vi "Model Initial Values - Add Inport RTM.vi"(8 "error in (no error)":errorcluster, 11 "Node Ptr":u64 format="%.0x") -> (0 "error out":errorcluster)   [LabVIEW 2011, in "Model Initial Values Custom Device.lvlib"]
uses:
  Model Initial Values Custom Device.lvlib
  <vilib>/NI Veristand/Custom Device API/Custom Device Item Ref.ctl
  NationalInstruments.VeriStand.SystemStorage
  Model Initial Values - Global.vi
  <vilib>/NI Veristand/Custom Device API/Get Item Property (Dependent Node Pointer).vi
  <vilib>/NI Veristand/Custom Device API/Set Item Property (Double Array).vi
  <vilib>/NI Veristand/Custom Device API/Set Item Property (String Array).vi
  <vilib>/NI Veristand/Custom Device API/Custom Device API.lvlib
  <vilib>/NI Veristand/Custom Device Tools/Custom Device Utility Library/Custom Device Utility Library.lvlib
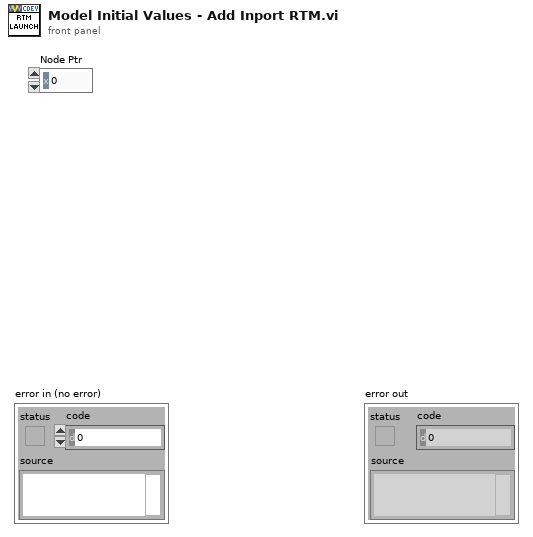
[diagram p1: front panel]
types:
  T1 = typedef "Custom Device API.lvlib/Custom Device Item Ref.ctl" = u64
  T2 = cluster{"MultipleSelection":bool, "ShowCheckBox":bool}
  T3 = typedef "Custom Device API.lvlib/Custom Device Item Info.ctl" = cluster{"Name":string, "Is Channel":bool, "GUID":string}
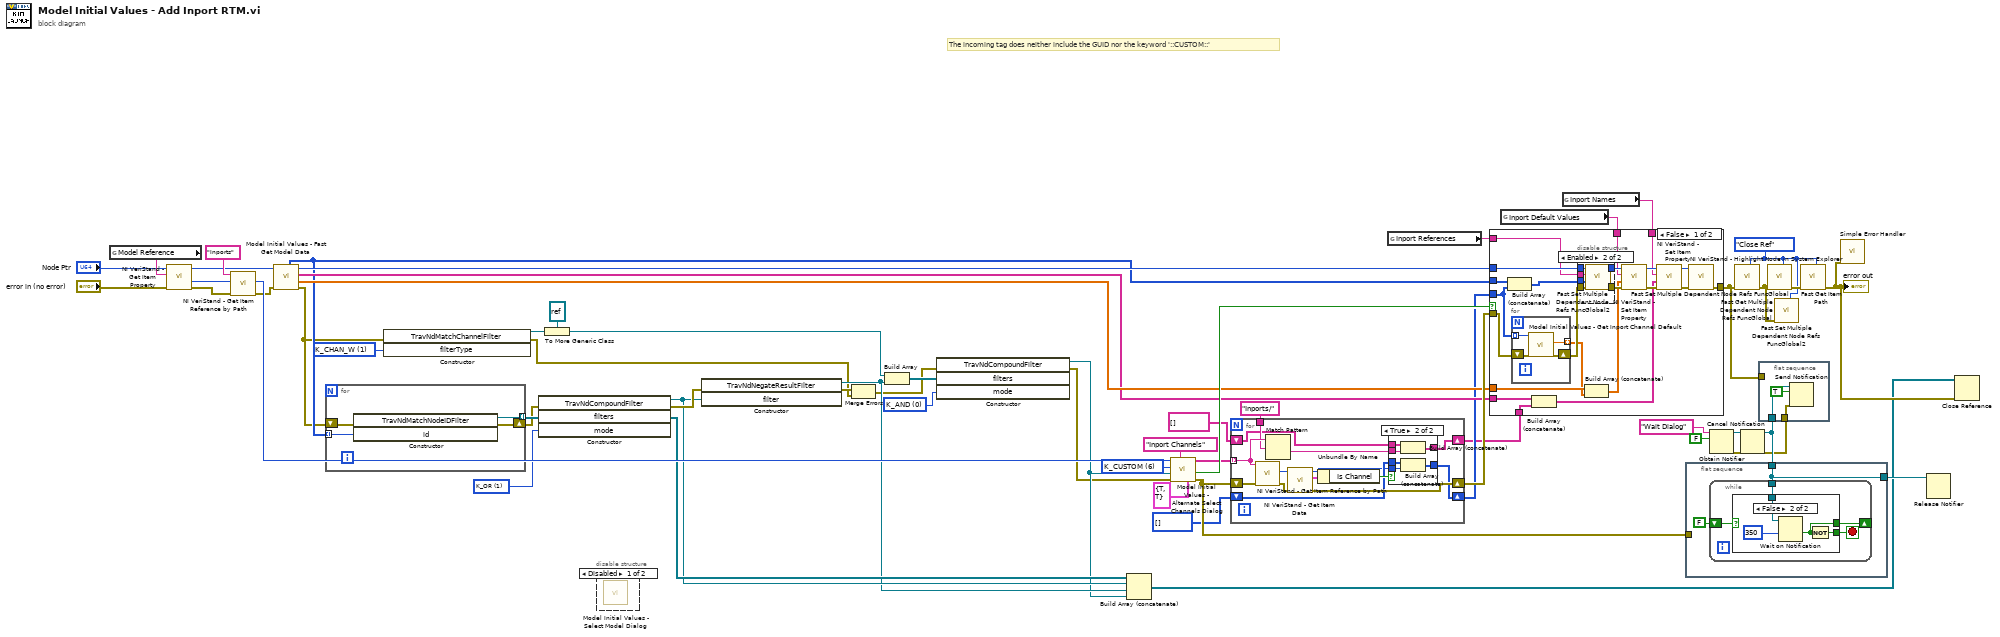
[diagram p0: block diagram]
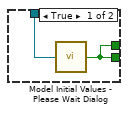
[diagram p3: hidden frame]
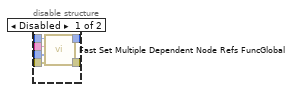
[diagram p5: hidden frame]
diagram:
  w13 = 0 items=["K_AND", "K_OR"] ("mode")
  w14 = u8 1 items=["K_CHAN_R", "K_CHAN_W", "K_CHAN_VOLT", "K_CHAN_FAULT"] ("filterType")
  w28 = 1 items=["K_AND", "K_OR"] ("mode")
  w2 = enum16{"Open or Add", "Close Ref"}."Close Ref" ("Action")
  w51 = u8 6 items=["K_CHAN_R", "K_CHAN_W", "K_CHAN_RW", "K_CHAN_VOLT", "K_CHAN_FAULT", "K_ALL", "K_CUSTOM"] ("Filter")
  # "The incoming tag does neither include the GUID nor the keyword '::CUSTOM::'"
  n1 = global read "Model Initial Values - Global.vi" "Model Reference"() -> (w59:string)
  n2 = call-poly <vilib>:"NI VeriStand - Get Item Property.vi"("error in (no error)"="error in (no error)", "Property Name"=w59, "Item Ref in"="Node Ptr") -> ("error out"=w55:errorcluster, "Dependent Node Ref"=w56:T1, "Item Ref out"=w42:T1)  [unwired: 5 in, 1 out]
  n3 = call <vilib>:"NI VeriStand - Get Item Reference by Path.vi"("error in (no error)"=w55, "Root Ref"=w56, "Item Path in"="Inports" ("Relative Item Path")) -> ("error out"=w41:errorcluster, "Item Ref"=w52:T1)  [unwired: 5 in, 2 out]
  n4 = call "Model Initial Values - Fast Get Model Data.vi"("error in (no error)"=w41, "Local Model Ref in"=w42) -> ("error out"=w6:errorcluster, "Inport Default Values"=w40:dbl[], "Inport Names"=w39:string[], "Local Model Ref out"=w60:T1, "Inport Refs"=w23:T1[])  [unwired: 4 in, 1 out]
  n5 = for {
    tunnel: [w64] -> w29 mode=indexing
    shift-right: [w63] -> w27
    shift-left: w6 -> [w62]
    tunnel: w23 -> [w61] mode=indexing
    n6 = constructor class="TravNdMatchNodeIDFilter"(error in=w62, "id"=w61) -> (reference out=w64:refnum<k24>, error out=w63:errorcluster)  [unwired: 2 in, 2 out]
  }
  n7 = constructor class="TravNdMatchChannelFilter"(error in=w6, "filterType"=w14) -> (reference out=w12:refnum<k24>, error out=w5:errorcluster)  [unwired: 2 in, 2 out]
  n8 = constructor class="TravNdCompoundFilter"(error in=w27, "filters"=w29, "mode"=w28) -> (reference out=w21:refnum<k24>, error out=w22:errorcluster, "filters"=w26:refnum<k24>[])  [unwired: 2 in, 2 out]
  n9 = To More Generic Class(target class=refnum<k24> refnum, reference=w12) -> (generic class reference=w10:refnum<k24>)
  n10 = disable-structure shown="Disabled" {
    frame Disabled {
      n11 = call "Model Initial Values - Select Model Dialog.vi"() -> ()  [unwired: 9 in, 3 out]
    }
    frame Enabled {
    }
  }
  n12 = constructor class="TravNdNegateResultFilter"(error in=w22, "filter"=w21) -> (reference out=w11:refnum<k24>, error out=w20:errorcluster)  [unwired: 2 in, 2 out]
  n13 = Merge Errors(w20, w5) -> (w4:errorcluster)
  n14 = Build Array(w10, w11) -> (w8:refnum<k24>[])
  n15 = constructor class="TravNdCompoundFilter"(error in=w4, "filters"=w8, "mode"=w13) -> (reference out=w7:refnum<k24>, error out=w3:errorcluster)  [unwired: 2 in, 3 out]
  n16 = Build Array (concatenate)(w26, w21, w11, w7) -> (w24:refnum<k24>[])
  n17 = call "Model Initial Values - Alternate Select Channels Dialog.vi"("Selection Properties"=T2 {"MultipleSelection"=TRUE, "ShowCheckBox"=TRUE}, "Channel Label"="Inport Channels", "error in (no error)"=w3, "Custom Filter"=w7, "Filter"=w51, "Start Item Ref"=w52) -> ("error out"=w44:errorcluster, "Canceled"=w48:bool, "Channel Paths"=w19:string[])  [unwired: 2 in, 1 out]
  n18 = for {
    tunnel: w19 -> [w77] mode=indexing
    shift-right: [w73] -> w50
    shift-left: w44 -> [w78]
    tunnel: "Inports/" ("Relative Item Path") -> [w76]
    shift-right: [w69] -> w15
    shift-left: string[] [] -> [w68]
    shift-right: [w65] -> w18
    shift-left: T1[] [] -> [w67]
    n19 = call <vilib>:"NI VeriStand - Get Item Reference by Path.vi"("error in (no error)"=w78, "Item Path in"=w77) -> ("error out"=w74:errorcluster, "Item Ref"=w75:T1)  [unwired: 6 in, 2 out]
    n20 = Match Pattern(string=w77, regular expression=w76) -> (after substring=w70:string)  [unwired: 1 in, 3 out]
    n21 = call <vilib>:"NI VeriStand - Get Item Data.vi"("error in (no error)"=w74, "Item Ref in"=w75) -> ("error out"=w73:errorcluster, "Item Info"=w72:T3, "Item Ref out"=w66:T1)  [unwired: 6 in, 1 out]
    n22 = Unbundle By Name(w72) -> ("Is Channel"=w71:bool)
    n23 = case shown="True" w71 {
      tunnel: w70 -> [_ w86]
      tunnel: [w80 w84] -> w69
      tunnel: w68 -> [w80 w85]
      tunnel: w67 -> [w79 w83]
      tunnel: w66 -> [_ w82]
      tunnel: [w79 w81] -> w65
      frame False {
      }
      frame True {
        n24 = Build Array (concatenate)(w85, w86) -> (w84:string[])
        n25 = Build Array (concatenate)(w83, w82) -> (w81:T1[])
      }
    }
  }
  n26 = global read "Model Initial Values - Global.vi" "Inport References"() -> (w58:string)
  n27 = global read "Model Initial Values - Global.vi" "Inport Default Values"() -> (w37:string)
  n28 = global read "Model Initial Values - Global.vi" "Inport Names"() -> (w38:string)
  n29 = case shown="False" w48 {
    tunnel: w18 -> [w90 _]
    tunnel: w23 -> [w108 _]
    tunnel: w50 -> [w89 w125]
    tunnel: w60 -> [w107 _]
    tunnel: [w104 w125] -> w43
    tunnel: w58 -> [w105 _]
    tunnel: w15 -> [w96 _]
    tunnel: w40 -> [w92 _]
    tunnel: w39 -> [w97 _]
    tunnel: w38 -> [w94 _]
    tunnel: w37 -> [w93 _]
    frame False {
      n30 = Build Array (concatenate)(w108, w90) -> (w106:T1[])
      n31 = for {
        tunnel: w90 -> [w124] mode=indexing
        shift-right: [w121] -> w88
        shift-left: w89 -> [w123]
        tunnel: [w122] -> w87 mode=indexing
        n32 = call "Model Initial Values - Get Inport Channel Default.vi"("error in"=w123, "Item Ref in"=w124) -> ("error out"=w121:errorcluster, "Default Value"=w122:dbl)  [unwired: 6 in, 1 out]
      }
      n33 = Build Array (concatenate)(w97, w96) -> (w95:string[])
      n34 = disable-structure shown="Enabled" {
        disable-tunnel: w107 -> [w114 w117]
        disable-tunnel: w106 -> [w113 w119]
        disable-tunnel: w105 -> [w112 w118]
        disable-tunnel: [w111 w116] -> w102
        disable-tunnel: [w110 w115] -> w101
        disable-tunnel: w88 -> [w109 w120]
        frame Disabled {
          n35 = call "Fast Set Multiple Dependent Node Refs FuncGlobal.vi"("error in (no error)"=w109, "Dependent Node Refs"=w113, "Base Property Name"=w112, "Item Ref in"=w114) -> ("error out"=w111:errorcluster, "Item Ref out"=w110:T1)  [unwired: 6 in]
        }
        frame Enabled {
          n36 = call "Fast Set Multiple Dependent Node Refs FuncGlobal2.vi"("error in (no error)"=w120, "Dependent Node Refs"=w119, "Base Property Name"=w118, "Item Ref in"=w117) -> ("error out"=w116:errorcluster, "Item Ref out"=w115:T1)  [unwired: 6 in]
        }
      }
      n37 = Build Array (concatenate)(w92, w87) -> (w91:dbl[])
      n38 = call-poly <vilib>:"NI VeriStand - Set Item Property.vi"("error in (no error)"=w102, "Value"=w91, "Property Name"=w93, "Item Ref in"=w101) -> ("error out"=w100:errorcluster, "Item Ref out"=w103:T1)  [unwired: 5 in, 1 out]
      n39 = call-poly <vilib>:"NI VeriStand - Set Item Property.vi"("error in (no error)"=w100, "Value"=w95, "Property Name"=w94, "Item Ref in"=w103) -> ("error out"=w99:errorcluster, "Item Ref out"=w98:T1)  [unwired: 5 in, 1 out]
      n40 = call <vilib>:"NI VeriStand - Highlight Node in System Explorer.vi"("error in (no error)"=w99, "Item Ref in"=w98) -> ("error out"=w104:errorcluster)  [unwired: 8 in, 1 out]
    }
    frame True {
    }
  }
  n41 = flat-sequence {
    tunnel: w44 -> [_]
    tunnel: w34 -> [w126]
    tunnel: [w126] -> w35
    frame #0 {
      n42 = while {
        tunnel: w126 -> [w130]
        shift-right: [w128] -> _
        shift-left: FALSE -> [w129]
        stop <- w131 stop-if-true
        n43 = case shown="False" w129 {
          tunnel: [w132 w135] -> w131
          tunnel: w130 -> [w133 w137]
          tunnel: [w132 w134] -> w128
          frame True {
            n44 = call "Model Initial Values - Please Wait Dialog.vi"("notifier out"=w133) -> ("Boolean"=w132:bool)
          }
          frame False {
            n45 = Wait on Notification(notifier=w137, timeout in ms (-1)=350) -> (timed out?=w134:bool)  [unwired: 2 in, 3 out]
            n46 = Not(x=w134) -> (.not. x?=w135:bool)
          }
        }
      }
    }
  }
  n47 = Obtain Notifier(name (unnamed)="Wait Dialog", notification data type=FALSE) -> (notifier out=w36:refnum<notifier>, error out=w32:errorcluster)  [unwired: 2 in, 1 out]
  n48 = call "Fast Get Multiple Dependent Node Refs FuncGlobal.vi"("Action"=w2, "error in (no error)"=w43) -> ("error out"=w1:errorcluster)  [unwired: 7 in, 2 out]
  n49 = Cancel Notification(0:w36, 3:w32) -> (8:w34:refnum<notifier>, 11:w33:errorcluster)  [unwired: 1 out]
  n50 = flat-sequence {
    tunnel: w34 -> [w140]
    tunnel: w33 -> [w139]
    tunnel: w43 -> [_]
    frame #0 {
      n51 = Send Notification(notification=TRUE, notifier=w140, error in (no error)=w139) -> ()  [unwired: 2 out]
    }
  }
  n52 = call "Fast Set Multiple Dependent Node Refs FuncGlobal.vi"("Action"=w2, "error in (no error)"=w1) -> ("error out"=w31:errorcluster)  [unwired: 8 in, 1 out]
  n53 = call "Fast Set Multiple Dependent Node Refs FuncGlobal2.vi"("Action"=w2, "error in (no error)"=w1) -> ()  [unwired: 8 in, 2 out]
  n54 = call "Fast Get Item Path.vi"("Action"=w2, "error in (no error)"=w31) -> ("error out"=w25:errorcluster)  [unwired: 6 in, 3 out]
  "error out" <- w25
  n55 = call <vilib>:"Simple Error Handler.vi"("error in (no error)"=w25) -> ()  [unwired: 4 in, 5 out]
  n56 = Release Notifier(notifier=w35) -> ()  [unwired: 2 in, 3 out]
  n57 = Close Reference(reference=w24, error in (no error)=w25) -> ()  [unwired: 1 out]
